vi "All Create Task.vi"(8 "error in":errorcluster, 10 "Config":T1={"AO config"=[], "AI config"=[], "DI config"=[], "DO config"=[], "TC config"=[{"Channel_Name"="", "Channel_Number"="", "Pre_Scale_min"=0.0, "Pre_Scale_max"=0.0, "units"=4, " type"=7}], "ACC config"=[], "SG config"=[], "Strain Gauge Settings"={"poisson ratio"=0.3, "nominal gage resistance"=120.0, "gage factor"=2.08}, "Bridge Settings"={"voltage excitation value"=3.3, "voltage excitation source"=10200, "initial bridge voltage"=0.0, "lead wire resistance"=1.7, "strain configuration"=10271}, "Sample Rate"={"AI Sample Rate"=0.0, "AO Sample Rate"=0.0, "DI Sample Rate"=0.0, "TC Sample Rate"=0.0, "DO Sample Rate"=0.0, "SG Sample Rate"=0.0, "ACC Sample Rate"=0.0}} {"Bridge Settings"."strain configuration" items=["Full Bridge I"=10183, "Full Bridge II"=10184, "Full Bridge III"=10185, "Half Bridge I"=10188, "Half Bridge II"=10189, "Quarter Bridge I"=10271, "Quarter Bridge II"=10272]; "Bridge Settings"."voltage excitation source" items=["Internal"=10200, "External"=10167, "None"=10230]; "ACC config"."Terminal configuration" items=["default"=-1, "RSE"=10083, "NRSE"=10078, "Differential"=10106, "Pseudodifferential"=12529]; "ACC config"."Sensitivity units" items=["mVolts/g"=12509, "Volts/g"=12510]; "TC config"."type" items=["J"=10072, "K"=10073, "N"=10077, "R"=10082, "S"=10085, "T"=10086, "B"=10047, "E"=10055]; "TC config"."units" items=["Deg C", "Deg F", "Kelvins", "Deg R", "From Custom Scale"]}, 11 "Task List":T3(array[ring])) -> (0 "error out":errorcluster, 3 "Task out":T2)   [LabVIEW 2022 SP3]
uses:
  Create Task/DI Create Task.vi
  Create Task/DO Create Task.vi
  Create Task/AO Create Task.vi
  Create Task/AI Create Task.vi
  Create Task/TC Create Task.vi
  Controls/Config.ctl
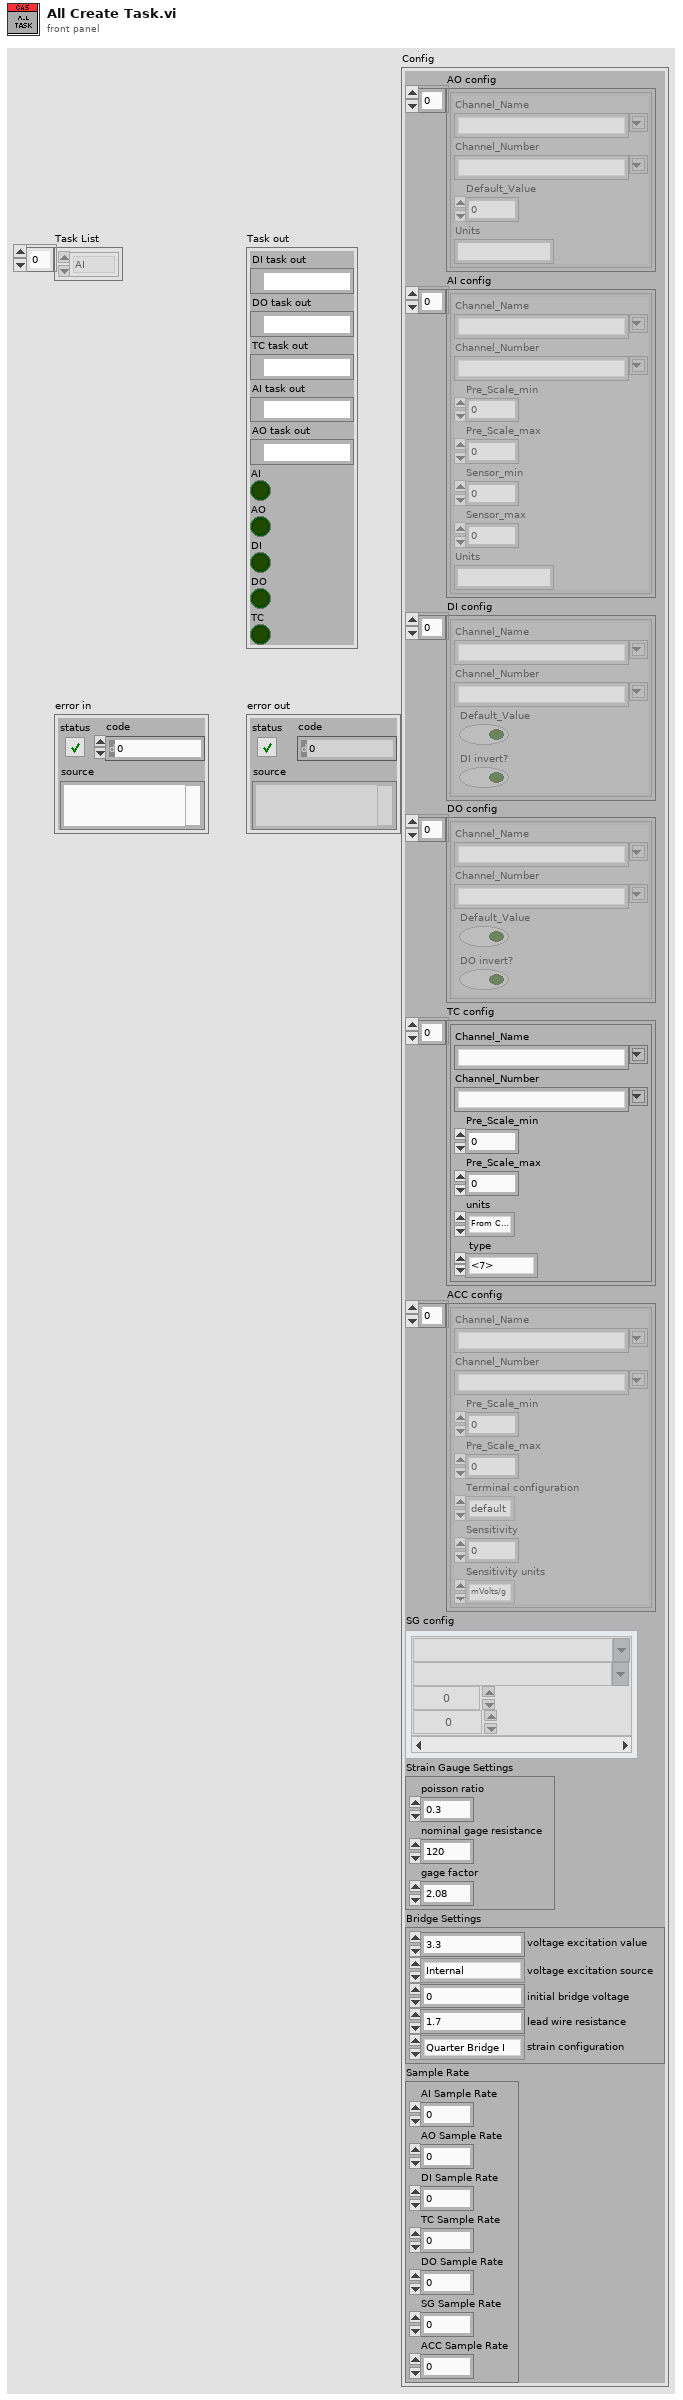
[diagram p1: front panel]
types:
  T1 = typedef "Config.ctl" = cluster{"AO config":cluster{"Channel_Name":string, "Channel_Number":string, "Default_Value":dbl, "Units":string}[], "AI config":cluster{"Channel_Name":string, "Channel_Number":string, "Pre_Scale_min":dbl, "Pre_Scale_max":dbl, "Sensor_min":dbl, "Sensor_max":dbl, "Units":string}[], "DI config":cluster{"Channel_Name":string, "Channel_Number":string, "Default_Value":bool, "DI invert?":bool}[], "DO config":cluster{"Channel_Name":string, "Channel_Number":string, "Default_Value":bool, "DO invert?":bool}[], "TC config":cluster{"Channel_Name":string, "Channel_Number":string, "Pre_Scale_min":dbl, "Pre_Scale_max":dbl, "units":i32, " type":i32}[], "ACC config":cluster{"Channel_Name":string, "Channel_Number":string, "Pre_Scale_min":dbl, "Pre_Scale_max":dbl, "Terminal configuration":i32, "Sensitivity":dbl, "Sensitivity units":i32}[], "SG config":cluster{"Channel_Name":string, "Channel_Number":string, "Pre_Scale_min":dbl, "Pre_Scale_max":dbl}[], "Strain Gauge Settings":cluster{"poisson ratio":dbl, "nominal gage resistance":dbl, "gage factor":dbl}, "Bridge Settings":cluster{"voltage excitation value":dbl, "voltage excitation source":i32, "initial bridge voltage":dbl, "lead wire resistance":dbl, "strain configuration":i32}, "Sample Rate":cluster{"AI Sample Rate":dbl, "AO Sample Rate":dbl, "DI Sample Rate":dbl, "TC Sample Rate":dbl, "DO Sample Rate":dbl, "SG Sample Rate":dbl, "ACC Sample Rate":dbl}}
  T2 = cluster{"DI task out":refnum<k21>, "DO task out":refnum<k21>, "TC task out":refnum<k21>, "AI task out":refnum<k21>, "AO task out":refnum<k21>, "AI":bool, "AO":bool, "DI":bool, "DO":bool, "TC":bool}
  T3 = enum16{"AI", "AO", "DI", "DO", "TC", "Strain", "ACC"}[]
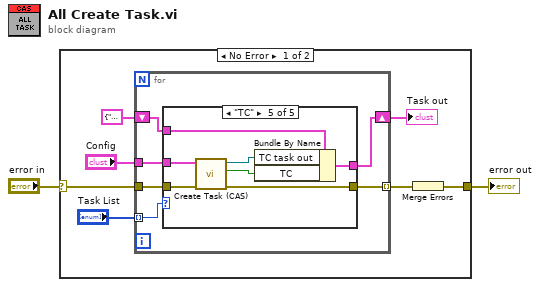
[diagram p0: block diagram]
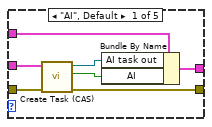
[diagram p2: hidden frame]
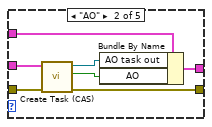
[diagram p3: hidden frame]
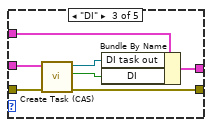
[diagram p4: hidden frame]
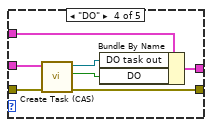
[diagram p5: hidden frame]
diagram:
  n1 = case shown="No Error" "error in" {
    selector: "error in" -> [w4 w51]
    tunnel: [w7 w51] -> w1
    frame No Error {
      n2 = for {
        tunnel: w4 -> [w15]
        tunnel: [w14] -> w8 mode=indexing
        tunnel: "Task List" -> [w13] mode=indexing
        shift-right: [w12] -> w6
        shift-left: T2 {"DI task out"="", "DO task out"="", "TC task out"="", "AI task out"="", "AO task out"="", "AI"=TRUE, "AO"=TRUE, "DI"=TRUE, "DO"=TRUE, "TC"=TRUE} ("Task out") -> [w11]
        tunnel: "Config" -> [w10]
        n3 = case shown="\"TC\"" w13 {
          tunnel: w15 -> [w22 w29 w36 w43 w50]
          tunnel: [w21 w28 w35 w42 w49] -> w14
          tunnel: [w20 w27 w34 w41 w48] -> w12
          tunnel: w11 -> [w19 w26 w33 w40 w47]
          tunnel: w10 -> [w16 w23 w30 w37 w44]
          frame "AI", Default {
            n4 = call-poly "Create Task (CAS).vi"("error in"=w22, "Config"=w16) -> ("error out"=w21:errorcluster, "empty?"=w17:bool, "AI Task"=w18:refnum<k21>)  [unwired: 7 in]
            n5 = Bundle By Name(cluster=w19, "AI task out"=w18, "AI"=w17) -> (w20:T2)
          }
          frame "AO" {
            n6 = call-poly "Create Task (CAS).vi"("error in"=w29, "Config"=w23) -> ("error out"=w28:errorcluster, "empty?"=w24:bool, "task out"=w25:refnum<k21>)  [unwired: 7 in]
            n7 = Bundle By Name(cluster=w26, "AO task out"=w25, "AO"=w24) -> (w27:T2)
          }
          frame "DI" {
            n8 = call-poly "Create Task (CAS).vi"("error in"=w36, "Config"=w30) -> ("error out"=w35:errorcluster, "empty?"=w31:bool, "DI Task"=w32:refnum<k21>)  [unwired: 7 in]
            n9 = Bundle By Name(cluster=w33, "DI task out"=w32, "DI"=w31) -> (w34:T2)
          }
          frame "DO" {
            n10 = call-poly "Create Task (CAS).vi"("error in"=w43, "Data"=w37) -> ("error out"=w42:errorcluster, "empty?"=w38:bool, "task out"=w39:refnum<k21>)  [unwired: 7 in]
            n11 = Bundle By Name(cluster=w40, "DO task out"=w39, "DO"=w38) -> (w41:T2)
          }
          frame "TC" {
            n12 = call-poly "Create Task (CAS).vi"("error in"=w50, "config"=w44) -> ("error out"=w49:errorcluster, "empty?"=w45:bool, "task out"=w46:refnum<k21>)  [unwired: 7 in]
            n13 = Bundle By Name(cluster=w47, "TC task out"=w46, "TC"=w45) -> (w48:T2)
          }
        }
      }
      "Task out" <- w6
      n14 = Merge Errors(w8) -> (w7:errorcluster)
    }
    frame Error {
    }
  }
  "error out" <- w1
